vi "_14_Sample_qsns_03[37].vi"() -> ()   [LabVIEW 2020]
panel:
  out "Waveform Graph":dbl[](graph)
  out "subarray":dbl[](array[numeric])
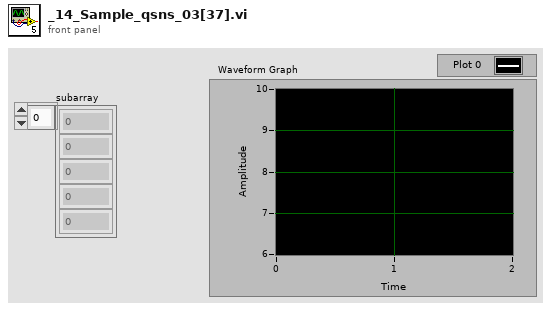
[diagram p1: front panel]
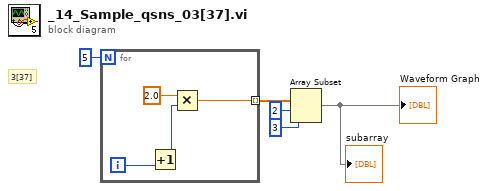
[diagram p0: block diagram]
diagram:
  # "3[37]"
  n1 = for {
    N: 5 -> [_]
    tunnel: [w6] -> w5 mode=indexing
    i -> [w8]
    n2 = Increment(x=w8) -> (x+1=w7:i32)
    n3 = Multiply(x=2.0, y=w7) -> (x*y=w6:dbl)
  }
  n4 = Array Subset(array=w5, index=2, length=3) -> (→"subarray" →"Waveform Graph":dbl[])
